vi "DAQ_Relay Control.vi"(0 "TSM Context Ref Num":T1, 5 "DAQ Relay":T2, 9 "Relay Action":T3, 11 "error in (no error)":errorcluster) -> (4 "TSM Context Ref Num Out":T1, 15 "error out":errorcluster)   [LabVIEW 2019]
uses:
  <vilib>/NI_TestStand_SemiconductorModule/NI_TestStand_Semiconductor_Module.lvlibp/PinMap/General/SemiconductorModuleContext.ctl
  Instrument Control/Relay - DAQmx/Pin Map/TSM DAQmx Relay Actions.ctl
  typedefs/DAQ_Relay.ctl
  Instrument Control/Relay - DAQmx/Pin Map/TSM DAQmx Relay.ctl
  Instrument Control/Relay - DAQmx/SubVIs/TSM DAQmx Relay Write.vi
  <vilib>/Utility/High Resolution Polling Wait.vi
  <vilib>/NI_TestStand_SemiconductorModule/NI_TestStand_Semiconductor_Module.lvlibp
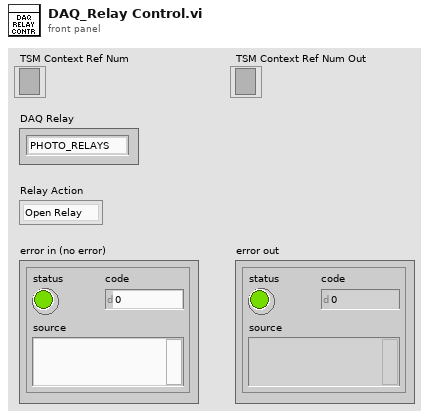
[diagram p1: front panel]
types:
  T1 = typedef "NI_TestStand_Semiconductor_Module.lvlibp/SemiconductorModuleContext.ctl" = refnum<k7>
  T2 = typedef "DAQ_Relay.ctl" = enum16{"PHOTO_RELAYS", "DAQ_U2", "DAQ_U3", "DAQ_U4", "DAQ_U6"}
  T3 = typedef "TSM DAQmx Relay Actions.ctl" = enum16{"Open Relay", "Close Relay"}
  T4 = typedef "TSM DAQmx Relay.ctl" = cluster{"TSM Context":T1, "Pins":tag[]}
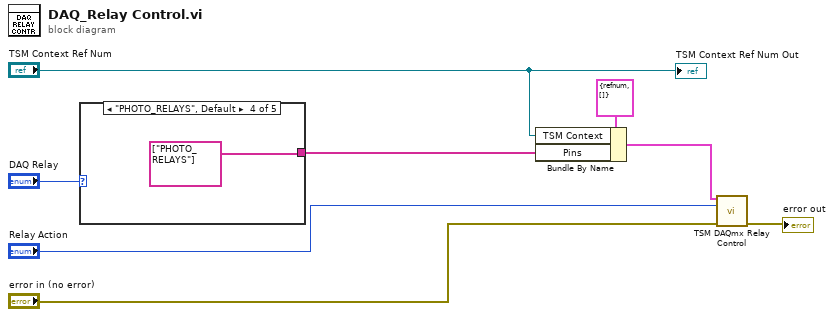
[diagram p0: block diagram]
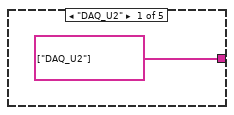
[diagram p2: hidden frame]
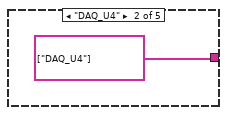
[diagram p3: hidden frame]
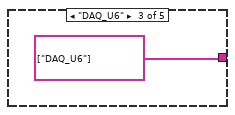
[diagram p4: hidden frame]
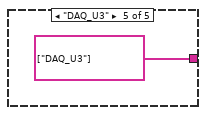
[diagram p5: hidden frame]
diagram:
  n1 = case shown="\"PHOTO_RELAYS\", Default" "DAQ Relay" {
    tunnel: [tag[] ["DAQ_U2"] ("Pins") tag[] ["DAQ_U4"] ("Pins") tag[] ["DAQ_U6"] ("Pins") tag[] ["PHOTO_RELAYS"] ("Pins") tag[] ["DAQ_U3"] ("Pins")] -> w1
    frame "DAQ_U2" {
    }
    frame "DAQ_U4" {
    }
    frame "DAQ_U6" {
    }
    frame "PHOTO_RELAYS", Default {
    }
    frame "DAQ_U3" {
    }
  }
  n2 = Bundle By Name(cluster=T4 {"TSM Context"=refnum, "Pins"=[]} ("TSM DAQmx Relay In"), "TSM Context"="TSM Context Ref Num", "Pins"=w1) -> (w3:T4)
  n3 = call "TSM DAQmx Relay Control.vi"("TSM DAQmx Relay In"=w3, "Relay Action"="Relay Action", "error in"="error in (no error)") -> ("error out"=→"error out":errorcluster)  [unwired: 12 in]
  "TSM Context Ref Num Out" <- "TSM Context Ref Num"
